vi "DAQmxSin INIT.vi"(7 "physical channels":tag="Dev2/ao0", 8 "error in":errorcluster, 10 "sine wave":dbl[](array[numeric]), 11 "DAQmxChannel":T1) -> (0 "error out":errorcluster, 3 "task out":refnum<k21>)   [LabVIEW 2020]
uses:
  <vilib>/DAQmx/write.llb/DAQmx Write (Analog Wfm 1Chan NSamp).vi
  <vilib>/DAQmx/create/channels.llb/DAQmx Create Channel (AO-Voltage-Basic).vi
  <vilib>/DAQmx/configure/timing.llb/DAQmx Timing (Sample Clock).vi
  <vilib>/DAQmx/miscellaneous.llb/DAQmx Fill In Error Info.vi
panel:
  out "number of samples written per channel":u32
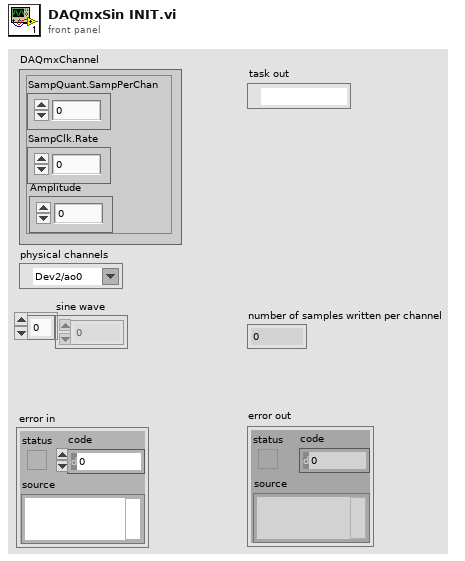
[diagram p1: front panel]
types:
  T1 = cluster{"SampClk.Rate":dbl, "SampQuant.SampPerChan":i32, "Amplitude":dbl}
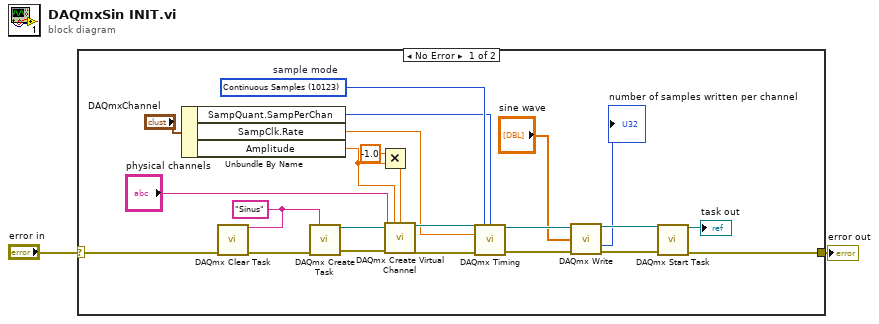
[diagram p0: block diagram]
diagram:
  n1 = case shown="No Error" "error in" {
    selector: "error in" -> [w16 w26]
    tunnel: [w24 w26] -> w2
    frame No Error {
      w14 = "Sinus" ("task name")
      w25 = 10123 items=["Finite Samples"=10178, "Continuous Samples"=10123, "Hardware Timed Single Point"=12522]  # sample mode
      n2 = Unbundle By Name("DAQmxChannel") -> ("SampQuant.SampPerChan"=w13:i32, "SampClk.Rate"=w12:dbl, "Amplitude"=w3:dbl)
      n3 = call <vilib>:"DAQmx Clear Task.vi"("task in"=w14, "error in"=w16) -> ("error out"=w15:errorcluster)  [unwired: 13 in]
      n4 = call <vilib>:"DAQmx Create Task.vi"("new task name"=w14, "error in"=w15) -> ("task out"=w21:refnum<k21>, "error out"=w18:errorcluster)  [unwired: 12 in]
      n5 = Multiply(x=-1.0, y=w3) -> (x*y=w5:dbl)
      n6 = call-poly <vilib>:"DAQmx Create Virtual Channel.vi"("task in"=w21, "maximum value"=w3, "minimum value"=w5, "physical channels"="physical channels", "error in"=w18) -> ("task out"=w20:refnum<k21>, "error out"=w19:errorcluster)  [unwired: 9 in]
      n7 = call-poly <vilib>:"DAQmx Timing.vi"("task/channels in"=w20, "sample mode"=w25, "samples per channel"=w13, "rate"=w12, "error in"=w19) -> ("task out"=w11:refnum<k21>, "error out"=w9:errorcluster)  [unwired: 9 in]
      n8 = call-poly <vilib>:"DAQmx Write.vi"("task/channels in"=w11, "data"="sine wave", "error in"=w9) -> ("task out"=w10:refnum<k21>, "number of samples written per channel"=→"number of samples written per channel":u32, "error out"=w8:errorcluster)  [unwired: 10 in]
      n9 = call <vilib>:"DAQmx Start Task.vi"("task/channels in"=w10, "error in"=w8) -> ("task out"=→"task out":refnum<k21>, "error out"=w24:errorcluster)  [unwired: 12 in]
    }
    frame Error {
    }
  }
  "error out" <- w2
